vi "SetParam.vi"(8 "error in (no error)":errorcluster caption="entrée d'erreur (pas d'erreur)", 10 "fowlkes_mallows_score":cluster{"sparse":bool}, 11 "Fowlkes_Mallows_Score.lvclass":refnum<class "Fowlkes_Mallows_Score.lvclass">) -> (0 "error out":errorcluster caption="sortie d'erreur", 3 "Fowlkes_Mallows_Score.lvclass":refnum<class "Fowlkes_Mallows_Score.lvclass">)   [LabVIEW 2020, in "Fowlkes_Mallows_Score.lvclass"]
doc: "Set Parameters"
uses:
  Fowlkes_Mallows_Score.lvclass
  Fowlkes_Mallows_Score.lvclass/Fowlkes_Mallows_Score.ctl
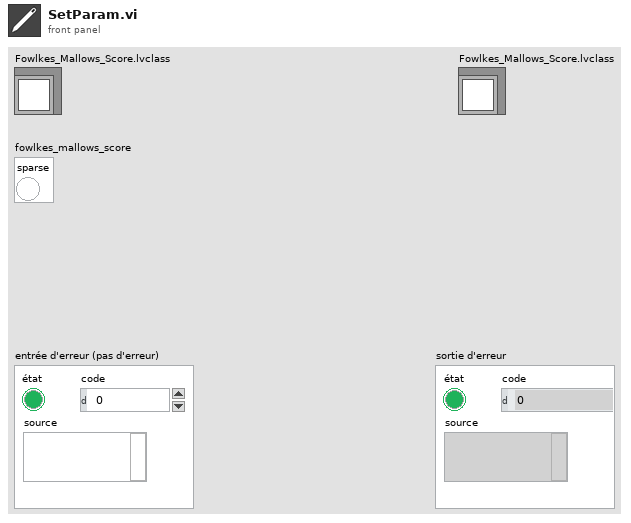
[diagram p1: front panel]
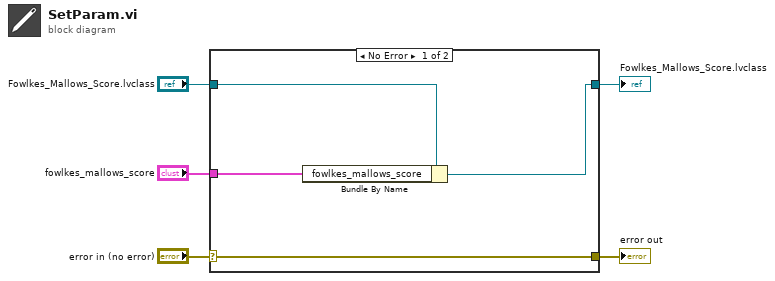
[diagram p0: block diagram]
diagram:
  n1 = case shown="No Error" "error in (no error)" {
    selector: "error in (no error)" -> [w9 w10]
    tunnel: [w9 w10] -> w4
    tunnel: [w7 w11] -> w2
    tunnel: "Fowlkes_Mallows_Score.lvclass" -> [w8 w11]
    tunnel: "fowlkes_mallows_score" -> [w6 _]
    frame No Error {
      n2 = Bundle By Name(cluster=w8, "fowlkes_mallows_score"=w6) -> (w7:refnum<class "Fowlkes_Mallows_Score.lvclass">)
    }
    frame Error {
    }
  }
  "error out" <- w4
  "Fowlkes_Mallows_Score.lvclass" <- w2
